vi "PRACTICA 3 INDICE DE MASA CORPORAL.vi"() -> ()   [LabVIEW 2017]
panel:
  in  "stop":bool
  in  "CENTIIMETROS":dbl
  out "Slide":dbl(slide) scale=10.0..40.0
  in  "ALTURA":dbl
  in  "PESO":dbl
  # "INDICE DE MASA CORPORAL"
  # "OBESIDAD"
  # "KG"
  # "M"
  # "SOBREPESO"
  # "PESO NORMAL"
  # "BAJO PESO"
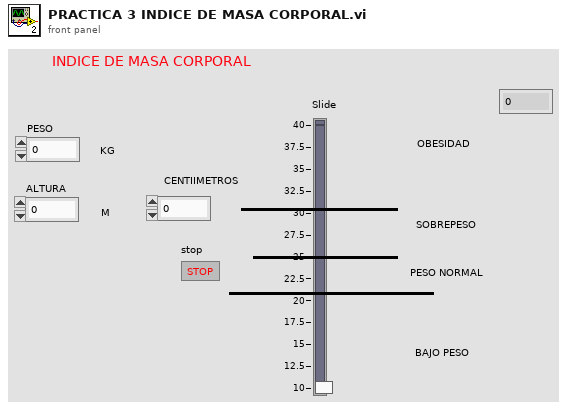
[diagram p1: front panel]
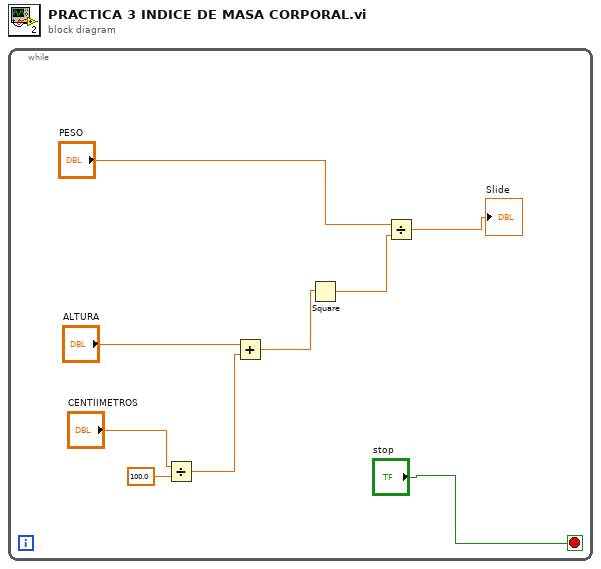
[diagram p0: block diagram]
diagram:
  n1 = while {
    stop <- "stop" stop-if-true
    n2 = Divide(x="CENTIIMETROS", y=100.0) -> (x/y=w3:dbl)
    n3 = Add(x="ALTURA", y=w3) -> (x+y=w8:dbl)
    n4 = Square(x=w8) -> (x^2=w6:dbl)
    n5 = Divide(x="PESO", y=w6) -> (x/y=→"Slide":dbl)
  }
